vi "Display NCL Logfile as CAN Frames.vi"() -> ()   [LabVIEW 2010]
doc: "This example demonstrates how to display the frames stored in a CAN Log File (*.NLC) and display them as NI-XNET CAN Frames."
uses:
  logfile.llb/XNET Logfile Mode.ctl
panel:
  in  "logfile path":path
  in  "Number of Frames to read (-1:all)":i32=-1
  out "Frames read":i32
  in  "Hexadecimal Display?":bool
  out "Frames":string[][](table)
  # "For instructions, select Help>>Show Context Help and drag your mouse over the VI icon on the top right."
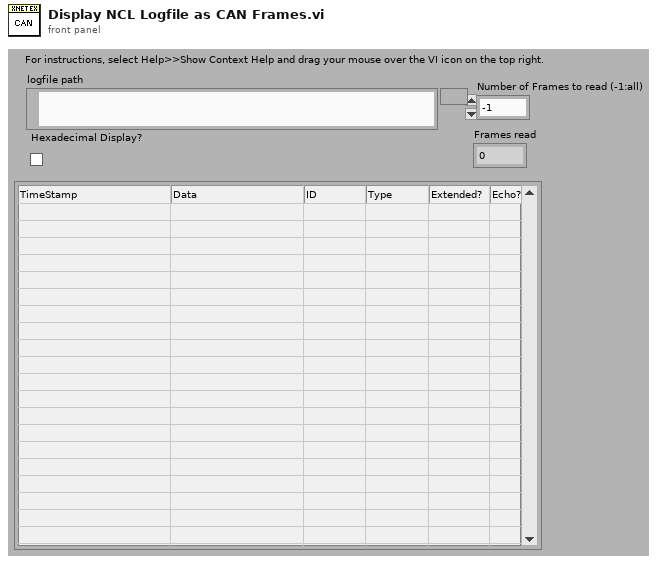
[diagram p1: front panel]
types:
  T1 = typedef "XNET Logfile Mode.ctl" = enum16{"Read", "Write (native endian)", "Write (big endian)"}
  T2 = typedef "XNET Logfile.ctl" = cluster{" file refnum":refnum<file>, "endian swap?":bool, "partial":u8[]}
  T3 = typedef "XNET Frame CAN.ctl" = cluster{"timestamp":timestamp, "payload":u8[], "identifier":u32, "type":T4, "extended?":bool, "echo?":bool}
  T4 = typedef "XNET Frame Type CAN.ctl" = u8
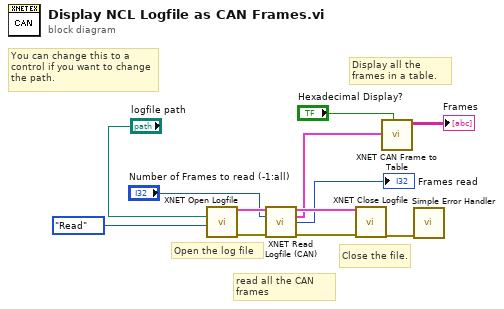
[diagram p0: block diagram]
diagram:
  # "You can change this to a control if you want to change the path."
  # "Close the file."
  # "Display all the frames in a table."
  # "read all the CAN frames"
  # "Open the log file"
  n1 = call "XNET Open Logfile.vi"("filepath"="logfile path", "mode"=XNET_Logfile_Mode."Read") -> ("logfile out"=w10:T2, "error out"=w9:errorcluster)  [unwired: 12 in]
  n2 = call "XNET Read Logfile (CAN).vi"("logfile in"=w10, "Maximum Number of Frames to read"="Number of Frames to read (-1:all)", "error in"=w9) -> ("logfile out"=w7:T2, "CAN frames"=w6:T3[], "Frames read"=→"Frames read":i32, "error out"=w8:errorcluster)  [unwired: 8 in, 1 out]
  n3 = call "XNET Close Logfile.vi"("logfile  in"=w7, "error in"=w8) -> ("error out"=w12:errorcluster)  [unwired: 12 in, 1 out]
  n4 = call "XNET CAN Frame to Table.vi"("Hexadecimal?"="Hexadecimal Display?", "CAN Frames (from XNET Read)"=w6) -> ("Output Array"=→"Frames":string[][])  [unwired: 9 in]
  n5 = call <vilib>:"Simple Error Handler.vi"("error in (no error)"=w12) -> ()  [unwired: 4 in, 5 out]
